vi "Test_ionizer_ps.vi"() -> ()   [LabVIEW 2016]
panel:
  in  "Ionizer VISA resource":refnum<visa-resource-name>="TCPIP0::192.168.1.160::966::SOCKET"
  in  "Loop multiple (ms)":u32=500
  out "Ionizer Iteration":i32
  out "Ionizer PS Current Actual 2":dbl
  out "Ionizer PS Current Actual":dbl(graph)
  out "Ionizer PS Voltage Actual 2":dbl
  out "Ionizer PS Voltage Actual":dbl(graph)
  out "Ionizer PS Current Set":dbl
  out "Ionizer PS Voltage Set":dbl
  out "Ionizer Error":errorcluster
  in  "stop":bool
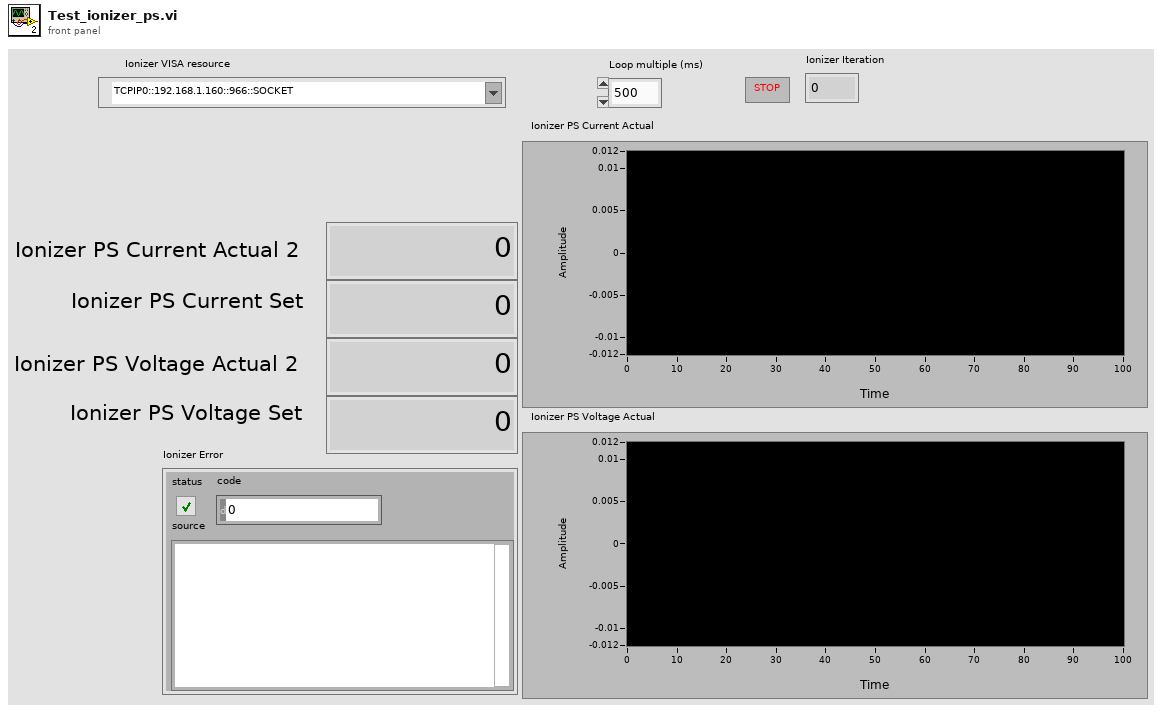
[diagram p1: front panel]
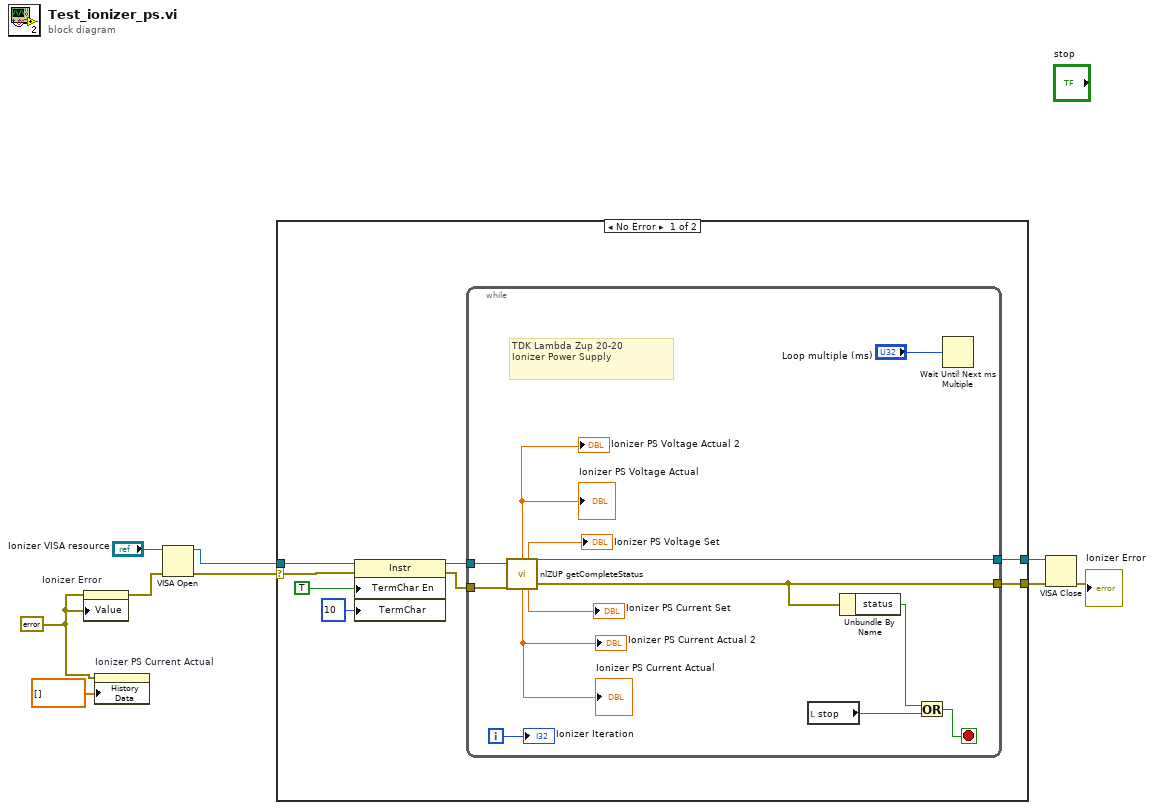
[diagram p0: block diagram]
diagram:
  w1 = errorcluster {"status"=FALSE, "code"=0, "source"=""} ("Ionizer Error")
  n1 = property on="Ionizer Error" class="Clust (strict)"(error in=w1, "Value"=w1) -> (error out=w5:errorcluster)  [unwired: 1 in, 1 out]
  n2 = property on="Ionizer PS Current Actual" class="WFChart (strict)"(error in=w1, "History Data"=dbl[] []) -> ()  [unwired: 1 in, 2 out]
  n3 = VISA Open(error in (no error)=w5, VISA resource name="Ionizer VISA resource") -> (VISA resource name=w9:refnum<visa-resource-name>, error out=w2:errorcluster)  [unwired: 3 in]
  n4 = case shown="No Error" w2 {
    selector: w2 -> [w10 w31]
    tunnel: w9 -> [w15 w32]
    tunnel: [w17 w32] -> w8
    tunnel: [w16 w31] -> w7
    frame No Error {
      n5 = property class="Instr"(reference=w15, error in=w10, "TermChar En"=TRUE ("Message Based Settings:Termination Character Enable"), "TermChar"=u8 10 ("Message Based Settings:Termination Character")) -> (reference out=w14:refnum<visa-resource-name>, error out=w13:errorcluster)
      n6 = while {
        tunnel: w14 -> [w25]
        tunnel: [w23] -> w17
        tunnel: w13 -> [w24]
        tunnel: [w22] -> w16
        i -> [w27]
        stop <- w28 stop-if-true
        # "TDK Lambda Zup 20-20\nIonizer Power Supply"
        n7 = call <instrlib>:"nlZUP getCompleteStatus.vi"("VISA resource name"=w25, "error in (no error)"=w24) -> ("Actual Voltage"=→"Ionizer PS Voltage Actual 2" →"Ionizer PS Voltage Actual":dbl, "Voltage Setting"=→"Ionizer PS Voltage Set":dbl, "VISA resource name out"=w23:refnum<visa-resource-name>, "Actual Current"=→"Ionizer PS Current Actual 2" →"Ionizer PS Current Actual":dbl, "Current Setting"=→"Ionizer PS Current Set":dbl, "error out"=w22:errorcluster)  [unwired: 5 in, 3 out]
        n8 = local read "stop"() -> (w26:bool)
        n9 = Unbundle By Name(w22) -> ("status"=w29:bool)
        n10 = Or(x=w29, y=w26) -> (x .or. y?=w28:bool)
        n11 = Wait Until Next ms Multiple(millisecond multiple="Loop multiple (ms)") -> ()  [unwired: 1 out]
        "Ionizer Iteration" <- w27
      }
    }
    frame Error {
    }
  }
  n12 = VISA Close(VISA resource name=w8, error in (no error)=w7) -> (error out=→"Ionizer Error":errorcluster)
